vi "VI Tree.vi"   [LabVIEW 2021, in "hashlib.lvlib"]
doc: "Hashlib VI Tree\n\nCreated by: Ryan Pacini"
uses:
  hashlib.lvlib
panel:
  # "SEE DIAGRAM\nFOR VI Tree"
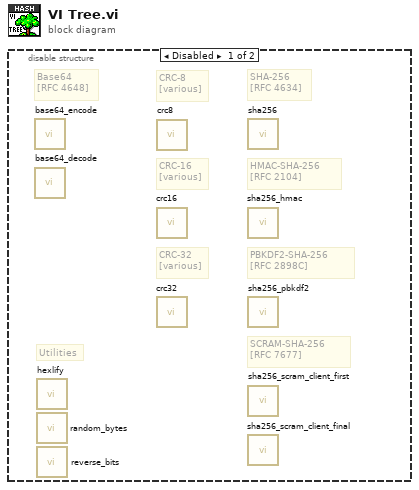
[diagram p0: block diagram]
diagram:
  n1 = disable-structure shown="Disabled" {
    frame Disabled {
      # "CRC-8\n[various]"
      # "Utilities"
      # "CRC-32\n[various]"
      # "CRC-16\n[various]"
      # "PBKDF2-SHA-256 \n[RFC 2898C]"
      # "SHA-256\n[RFC 4634]"
      # "HMAC-SHA-256\n[RFC 2104]"
      # "SCRAM-SHA-256 \n[RFC 7677]"
      # "Base64\n[RFC 4648]"
      n2 = call "base64_encode.vi"() -> ()  [unwired: 11 in, 1 out]
      n3 = call "base64_decode.vi"() -> ()  [unwired: 11 in, 1 out]
      n4 = call "hexlify.vi"() -> ()  [unwired: 11 in, 1 out]
      n5 = call "random_bytes.vi"() -> ()  [unwired: 11 in, 1 out]
      n6 = call "reverse_bits.vi"() -> ()  [unwired: 11 in, 1 out]
      n7 = call "crc8.vi"() -> ()  [unwired: 11 in, 1 out]
      n8 = call "crc16.vi"() -> ()  [unwired: 11 in, 1 out]
      n9 = call "crc32.vi"() -> ()  [unwired: 11 in, 1 out]
      n10 = call "sha256.vi"() -> ()  [unwired: 11 in, 1 out]
      n11 = call "sha256_hmac.vi"() -> ()  [unwired: 11 in, 1 out]
      n12 = call "sha256_pbkdf2.vi"() -> ()  [unwired: 11 in, 1 out]
      n13 = call "sha256_scram_client_first.vi"() -> ()  [unwired: 11 in, 1 out]
      n14 = call "sha256_scram_client_final.vi"() -> ()  [unwired: 11 in, 1 out]
    }
    frame Enabled {
    }
  }
